vi "Set Trigger.vi"(3 "burst count":i32=2 min=2 max=32766, 4 "burst period":i32=4 min=4 max=32766, 5 "Trigger Slope":bool, 6 "internal/burst trigger rate":dbl=0.001 min=0.001 max=1000000.0 format="%.3f", 7 "Input Impedance":bool, 8 "error in (no error)":errorcluster, 9 "external trigger level":sgl=1.0 min=-2.56 max=2.56 format="%.2f", 10 "Trigger Mode":T1, 11 "VISA Refnum in":refnum<visa-resource-name>) -> (0 "error out":errorcluster)   [LabVIEW 2012, in "SRS_DG535_Lib.lvlib"]
uses:
  SRS_DG535_Lib.lvlib
  Command/DG535_TriggerMode.ctl
panel:
  out "output string 2":string
  out "output string":string
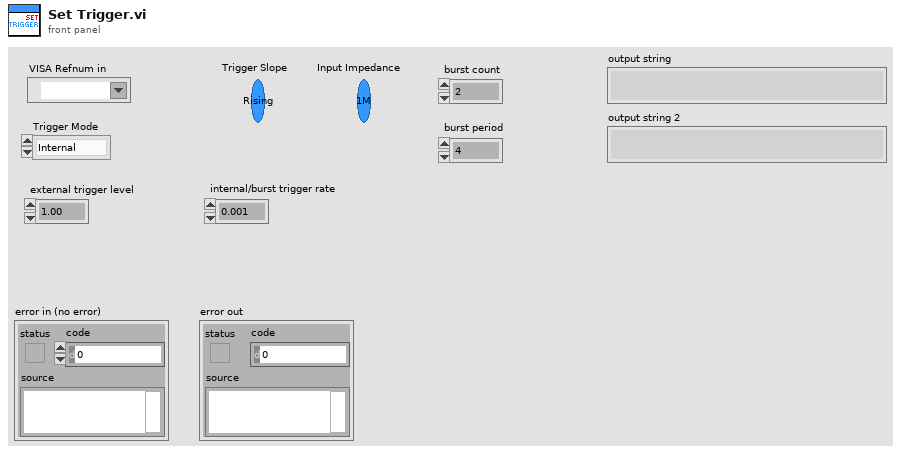
[diagram p1: front panel]
types:
  T1 = typedef "SRS_DG535_Lib.lvlib/DG535_TriggerMode.ctl" = enum16{"Internal", "External", "SingleShot", "Burst", "Line"}
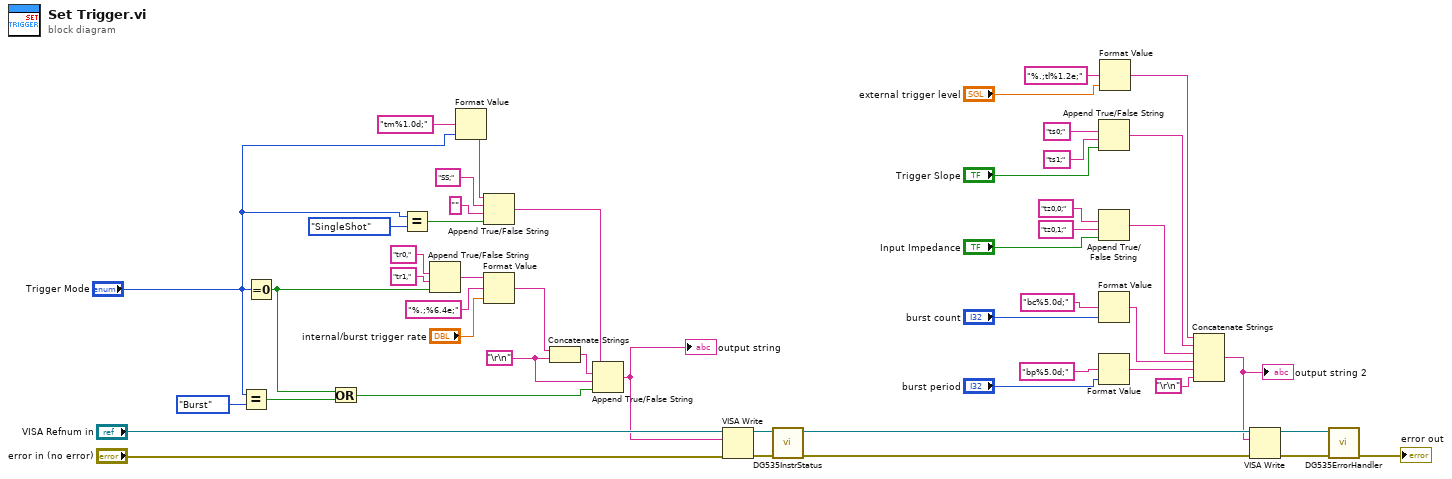
[diagram p0: block diagram]
diagram:
  w1 = "\r\n"
  n1 = Equal?(x="Trigger Mode", y=DG535_TriggerMode."Burst") -> (x = y?=w43:bool)
  n2 = Equal To 0?(x="Trigger Mode") -> (x = 0?=w45:bool)
  n3 = Or(x=w45, y=w43) -> (x .or. y?=w44:bool)
  n4 = Equal?(x="Trigger Mode", y=DG535_TriggerMode."SingleShot") -> (x = y?=w48:bool)
  n5 = Append True/False String(1:w45, 2:"tr1,", 3:"tr0,") -> (0:w38:string)  [unwired: 1 in]
  n6 = Format Value(format string="tm%1.0d;", value (0)="Trigger Mode") -> (output string=w2:string)  [unwired: 1 in]
  n7 = Append True/False String(1:w48, 2:"", 3:"SS;", 4:w2) -> (0:w3:string)
  n8 = Format Value(string ("")=w38, format string="%.;%6.4e;", value (0)="internal/burst trigger rate") -> (output string=w4:string)
  n9 = Concatenate Strings(w4, w1) -> (w7:string)
  n10 = Append True/False String(1:w44, 2:w1, 3:w7, 4:w3) -> (0:w20:string)
  "output string" <- w20
  n11 = VISA Write(VISA resource name="VISA Refnum in", write buffer=w20, error in (no error)="error in (no error)") -> (VISA resource name out=w17:refnum<visa-resource-name>, error out=w19:errorcluster)  [unwired: 1 out]
  n12 = call "DG535InstrStatus.vi"("error in"=w19, "VISA resource name"=w17) -> ("error out"=w18:errorcluster, "duplicate VISA resource"=w16:refnum<visa-resource-name>)  [unwired: 7 in, 1 out]
  n13 = Append True/False String(1:"Trigger Slope", 2:"ts1;", 3:"ts0;") -> (0:w9:string)  [unwired: 1 in]
  n14 = Append True/False String(1:"Input Impedance", 2:"tz0,1;", 3:"tz0,0;") -> (0:w10:string)  [unwired: 1 in]
  n15 = Format Value(format string="bc%5.0d;", value (0)="burst count") -> (output string=w11:string)  [unwired: 1 in]
  n16 = Format Value(format string="bp%5.0d;", value (0)="burst period") -> (output string=w12:string)  [unwired: 1 in]
  n17 = Format Value(format string="%.;tl%1.2e;", value (0)="external trigger level") -> (output string=w8:string)  [unwired: 1 in]
  n18 = Concatenate Strings(w8, w9, w10, w11, w12, "\r\n") -> (w13:string)
  "output string 2" <- w13
  n19 = VISA Write(VISA resource name=w16, write buffer=w13, error in (no error)=w18) -> (VISA resource name out=w14:refnum<visa-resource-name>, error out=w15:errorcluster)  [unwired: 1 out]
  n20 = call "DG535ErrorHandler.vi"("error in"=w15, "VISA resource name"=w14) -> ("error out"=→"error out":errorcluster)  [unwired: 7 in, 2 out]
